vi "East.vi"(9 "Spheres in":cluster{i32, i32}[](array[cluster]), 10 "Cubes":cluster{i32, i32}[](array[cluster]), 11 "Eastmost":i32) -> (1 "Spheres out":cluster{i32, i32}[](array[cluster]))   [LabVIEW 2023, in "d14.lvlib"]
uses:
  d14.lvlib
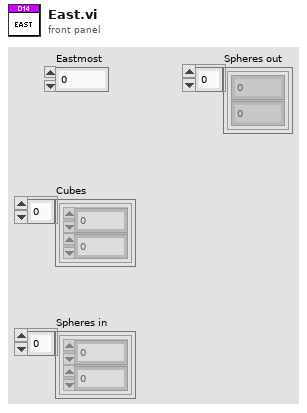
[diagram p1: front panel]
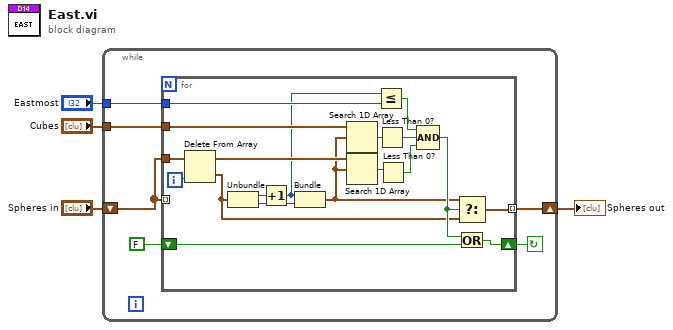
[diagram p0: block diagram]
diagram:
  n1 = while {
    tunnel: "Cubes" -> [w10]
    shift-right: [w9] -> w4
    shift-left: "Spheres in" -> [w5]
    tunnel: "Eastmost" -> [w8]
    stop <- w6 continue-if-true
    n2 = for {
      tunnel: w10 -> [w29]
      tunnel: w5 -> [_] mode=indexing
      tunnel: [w26] -> w9 mode=indexing
      tunnel: w8 -> [w25]
      shift-right: [w20] -> w6
      shift-left: FALSE ("x .and. y?") -> [w21]
      tunnel: w5 -> [w19]
      i -> [w17]
      n3 = Delete From Array(array=w19, index=w17) -> (deleted portion=w16:cluster{i32, i32}, array with subset deleted=w18:cluster{i32, i32}[])  [unwired: 1 in]
      n4 = Unbundle(w16) -> (w28:i32, w12:i32)
      n5 = Increment(x=w28) -> (x+1=w11:i32)
      n6 = Bundle(w11, w12) -> (w15:cluster{i32, i32})  [unwired: 1 in]
      n7 = Search 1D Array(1D array=w29, element=w15) -> (index of element=w27:i32)  [unwired: 1 in]
      n8 = Search 1D Array(1D array=w18, element=w15) -> (index of element=w14:i32)  [unwired: 1 in]
      n9 = Less Or Equal?(x=w11, y=w25) -> (x <= y?=w24:bool)
      n10 = Less Than 0?(x=w27) -> (x < 0?=w23:bool)
      n11 = Less Than 0?(x=w14) -> (x < 0?=w13:bool)
      n12 = Compound Arithmetic op=AND(w24, w23, w13) -> (w22:bool)
      n13 = Select(t=w15, s=w22, f=w16) -> (s? t:f=w26:cluster{i32, i32})
      n14 = Or(x=w22, y=w21) -> (x .or. y?=w20:bool)
    }
  }
  "Spheres out" <- w4
